vi "Search Array.vi"(4 "error in (no error)":errorcluster, 5 "Searchable Property (Name)":T1, 6 "Search Value":variant, 7 "Controller Array in":refnum<class "Controller Array.lvclass">) -> (0 "error out":errorcluster, 1 "Controller found":refnum<class "Generic Plugin.lvclass">, 2 "Index of found":i32, 3 "Controller Array out":refnum<class "Controller Array.lvclass">)   [LabVIEW 2020, in "Controller Array.lvclass"]
doc: "Search the array of controllers for the specified Searchable Property, using the Search Value by casting it to the type of the Searchable Property. This VI will only return the first occurance. If no element was found, it returns an index of -1 and a generic controller object."
uses:
  Controller Array.lvclass
  Controller/Generic Plugin.lvclass
  Controller/Controller Type.ctl
  Searchable Properties.ctl
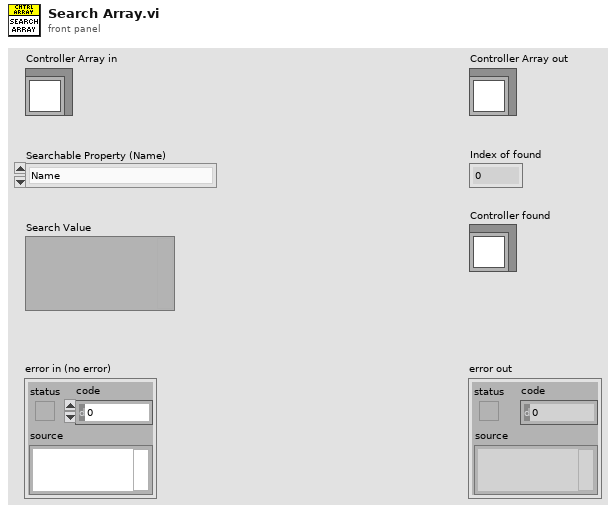
[diagram p1: front panel]
types:
  T1 = typedef "Controller Array.lvclass/Searchable Properties.ctl" = enum16{"Name", "Controller Type"}
  T2 = typedef "Generic Plugin.lvclass/Controller Type.ctl" = enum16{"Invalid", "Temperature Controller", "Pump Controller", "Generic Optimizer", "LC Parser"}
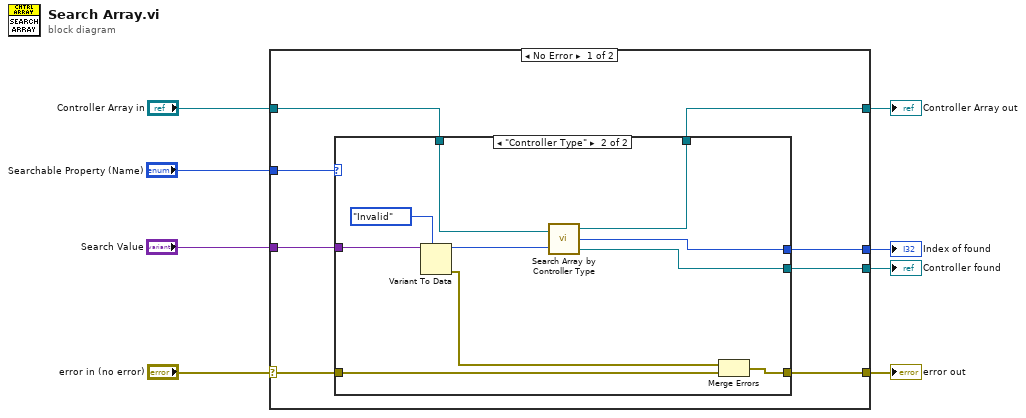
[diagram p0: block diagram]
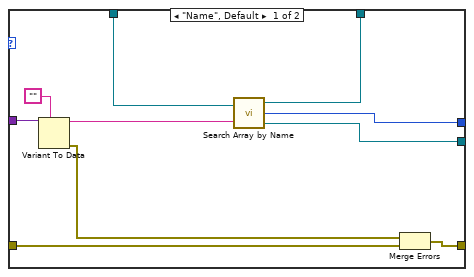
[diagram p2: hidden frame]
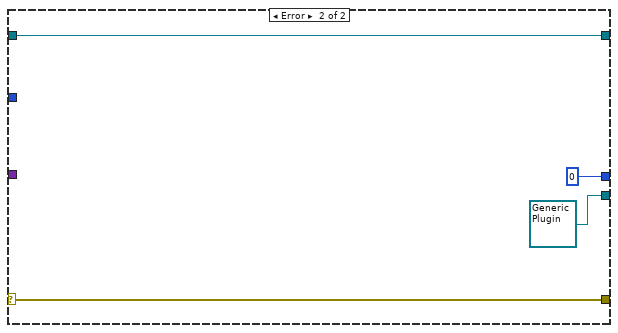
[diagram p3: hidden frame]
diagram:
  n1 = case shown="No Error" "error in (no error)" {
    selector: "error in (no error)" -> [w14 w40]
    tunnel: [w13 w40] -> w7
    tunnel: [w9 w39] -> w6
    tunnel: "Controller Array in" -> [w10 w39]
    tunnel: "Searchable Property (Name)" -> [w16 _]
    tunnel: "Search Value" -> [w15 _]
    tunnel: [w12 refnum<class "Generic Plugin.lvclass"> refnum ("Controller.lvclass")] -> w3
    tunnel: [w11 0] -> w2
    frame No Error {
      n2 = case shown="\"Controller Type\"" w16 {
        tunnel: w15 -> [w26 w36]
        tunnel: w14 -> [w22 w34]
        tunnel: [w23 w33] -> w13
        tunnel: [w19 w29] -> w9
        tunnel: [w17 w27] -> w12
        tunnel: [w18 w28] -> w11
        tunnel: w10 -> [w21 w30]
        frame "Name", Default {
          n3 = Variant To Data(type="", Variant=w26) -> (data=w20:string, error out=w24:errorcluster)  [unwired: 1 in]
          n4 = call "Search Array by Name.vi"("Controller Array in"=w21, "Name"=w20) -> ("Controller Array Out"=w19:refnum<class "Controller Array.lvclass">, "Index of found"=w18:i32, "Controller found"=w17:refnum<class "Generic Plugin.lvclass">)
          n5 = Merge Errors(w24, w22) -> (w23:errorcluster)
        }
        frame "Controller Type" {
          n6 = Variant To Data(type=Controller_Type."Invalid" ("Controller Type"), Variant=w36) -> (data=w31:T2, error out=w32:errorcluster)  [unwired: 1 in]
          n7 = call "Search Array by Controller Type.vi"("Controller Array in"=w30, "Controller Type"=w31) -> ("Controller Array Out"=w29:refnum<class "Controller Array.lvclass">, "Index of found"=w28:i32, "Controller found"=w27:refnum<class "Generic Plugin.lvclass">)
          n8 = Merge Errors(w32, w34) -> (w33:errorcluster)
        }
      }
    }
    frame Error {
    }
  }
  "error out" <- w7
  "Controller Array out" <- w6
  "Controller found" <- w3
  "Index of found" <- w2
